vi "DSF.Execution.Builder.Get Plugin Buffer Pool.vi"(8 "error in (no error)":errorcluster, 10 "plugin id":i32, 11 "Builder in":refnum<class "DSF.Execution.Builder.lvclass">) -> (0 "error out":errorcluster, 2 "BufferPool":refnum<class "DSF.Memory.BufferPool.lvclass">, 3 "Builder out":refnum<class "DSF.Execution.Builder.lvclass">)   [LabVIEW 2016, in "DSF.Execution.lvlib" / "DSF.Execution.Builder.lvclass"]
uses:
  DSF.Execution.Builder.lvclass
  Memory.BufferPool/DSF.Memory.BufferPool.lvclass
  DSF.Execution.Builder.lvclass/DSF.Execution.Builder.ctl
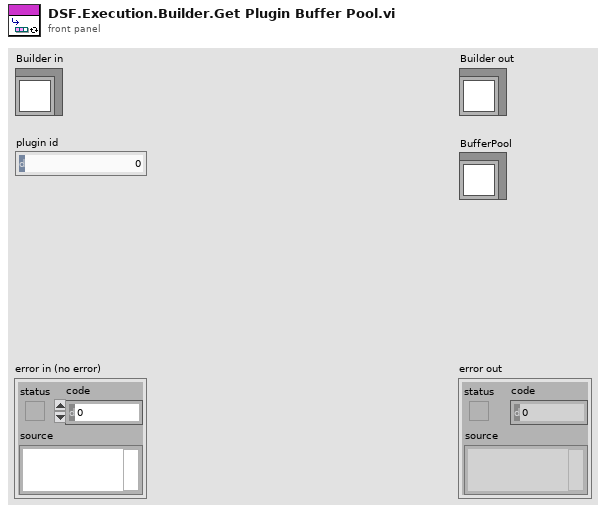
[diagram p1: front panel]
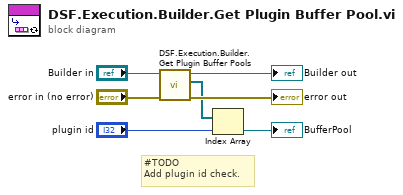
[diagram p0: block diagram]
diagram:
  # "#TODO\nAdd plugin id check."
  n1 = call "DSF.Execution.Builder.Get Plugin Buffer Pools.vi"("error in (no error)"="error in (no error)", "Builder in"="Builder in") -> ("error out"=→"error out":errorcluster, "Plugin Buffer Pools"=w3:refnum<class "DSF.Memory.BufferPool.lvclass">[], "Builder out"=→"Builder out":refnum<class "DSF.Execution.Builder.lvclass">)  [unwired: 7 in]
  n2 = Index Array(array=w3, index="plugin id") -> (element=→"BufferPool":refnum<class "DSF.Memory.BufferPool.lvclass">)
